vi "Script Custom Device.vi"(8 "error in":errorcluster, 9 "Hardware Configuration File Path":path, 10 "Parameters Configuration File Path":path, 11 "System Definition File Path In":path) -> (0 "error out":errorcluster, 1 "Ballard ARINC 429 custom device out":T1 format="%.0x", 2 "System Definition Reference":refnum<k24>, 3 "System Definition File Path Out":path)   [LabVIEW 2020]
uses:
  NationalInstruments.VeriStand.SystemDefinitionAPI
  <vilib>/NI VeriStand/Custom Device API/Custom Device Item Ref.ctl
  Shared/Device Parameters.ctl
  Shared/Initialization Method.ctl
  niveristand-custom-device-testing-tools/VeriStandTestUtilities/VeriStandTestUtilities.lvlib
  Scripting/Ballard/Ballard ARINC 429 Scripting.lvlib
  <vilib>/NI VeriStand/Custom Device API/Custom Device API.lvlib
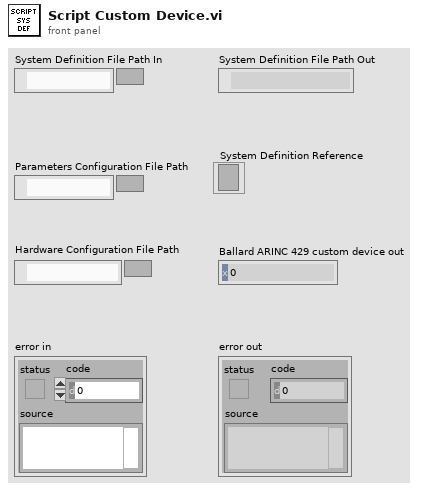
[diagram p1: front panel]
types:
  T1 = typedef "Custom Device API.lvlib/Custom Device Item Ref.ctl" = u64
  T2 = typedef "Device Parameters.ctl" = cluster{"initialization method":T3, "card number":i32, "PXI slot number":i32, "core number":i32}
  T3 = typedef "Initialization Method.ctl" = enum16{"PXI Slot Number", "Card Number"}
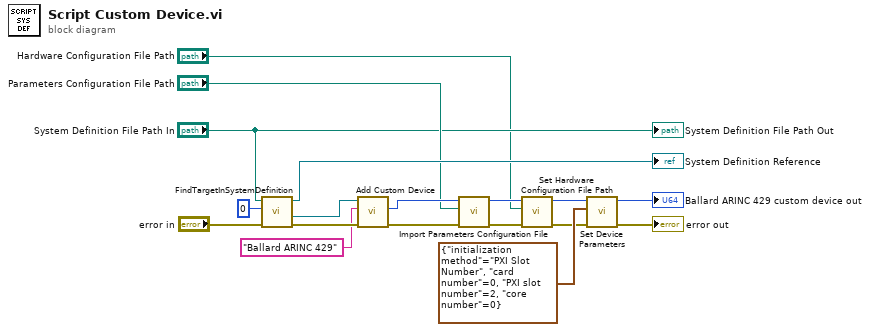
[diagram p0: block diagram]
diagram:
  n1 = call "FindTargetInSystemDefinition.vi"("error in"="error in", "target index"=0 ("index"), "system definition path"="System Definition File Path In") -> ("error out"=w17:errorcluster, "Target"=w16:refnum<k24>, "System Definition"=→"System Definition Reference":refnum<k24>)  [unwired: 5 in, 1 out]
  n2 = call "Add Custom Device.vi"("error in"=w17, "name"="Ballard ARINC 429", "target in"=w16) -> ("error out"=w11:errorcluster, "Ballard ARINC 429 custom device"=w10:T1)  [unwired: 6 in, 1 out]
  n3 = call "Import Parameters Configuration File.vi"("error in"=w11, "parameters configuration file path"="Parameters Configuration File Path", "Ballard ARINC 429 custom device in"=w10) -> ("error out"=w5:errorcluster, "Ballard ARINC 429 custom device out"=w3:T1)  [unwired: 7 in]
  n4 = call "Set Hardware Configuration File Path.vi"("error in"=w5, "hardware configuration file path"="Hardware Configuration File Path", "Ballard ARINC 429 custom device in"=w3) -> ("error out"=w4:errorcluster, "Ballard ARINC 429 custom device out"=w2:T1)  [unwired: 7 in]
  n5 = call "Set Device Parameters.vi"("error in"=w4, "device parameters"=T2 {"initialization method"=enum."PXI Slot Number", "card number"=0, "PXI slot number"=2, "core number"=0}, "Ballard ARINC 429 custom device in"=w2) -> ("error out"=→"error out":errorcluster, "Ballard ARINC 429 custom device out"=→"Ballard ARINC 429 custom device out":T1)  [unwired: 7 in]
  "System Definition File Path Out" <- "System Definition File Path In"
